vi "Example - Set Menu Items.vi"(8 "Error In":errorcluster, 10 "MenuHierarchyPaths":string[](array[string])=["Edit:Copy", "Edit:Paste", "Tools:Build", "Tools:Advanced:Mass Compile", "Tools:Advanced:Clear Cache"], 11 "Button":bool) -> (0 "Error Out":errorcluster)   [LabVIEW 2016, in "SLL Menu.lvlib"]
doc: "Example for Set Menu Items which builds a hierarchical run-time shortcut menu from colon-delimited paths."
uses:
  SLL Menu.lvlib
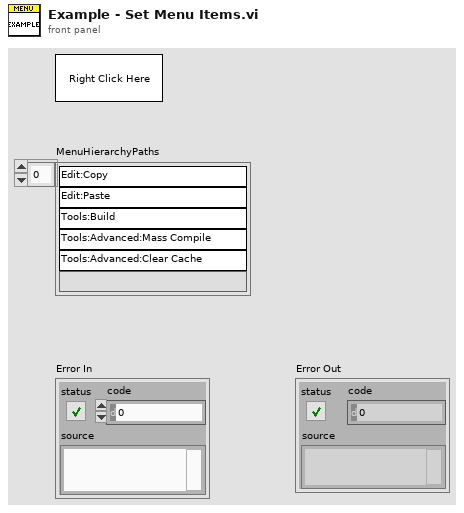
[diagram p1: front panel]
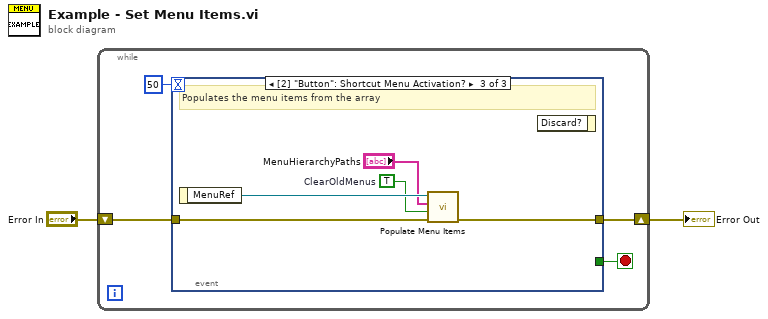
[diagram p0: block diagram]
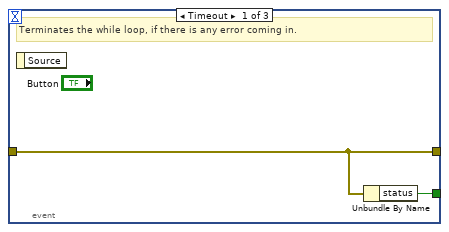
[diagram p2: hidden frame]
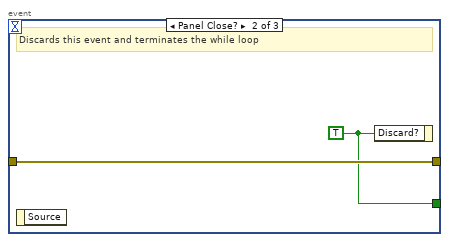
[diagram p3: hidden frame]
diagram:
  n1 = while {
    shift-right: [w3] -> w1
    shift-left: "Error In" -> [w4]
    stop <- w5 stop-if-true
    n2 = event shown="[2] \"Button\": Shortcut Menu Activation?" {
      selector: _ -> [_ _ _]
      dyn-events: _ -> [_ _ _]
      timeout: 50 -> [_ _ _]
      tunnel: [w7 w9 _] -> w5
      tunnel: w4 -> [w8 w10 w15]
      tunnel: [w8 w10 w13] -> w3
      event Timeout {
        # "Terminates the while loop, if there is any error coming in."
        n3 = event-data() -> ()  [unwired: 1 in, 1 out]
        n4 = Unbundle By Name(w8) -> ("status"=w7:bool)
      }
      event Panel Close? {
        w9 = TRUE ("Discard?")
        # "Discards this event and terminates the while loop"
        n5 = event-data() -> ()  [unwired: 1 in, 1 out]
        n6 = event-data("Discard?"=w9) -> ()  [unwired: 1 in, 1 out]
      }
      event "Button": Shortcut Menu Activation? {
        w11 = TRUE  # ClearOldMenus
        # "Populates the menu items from the array"
        n7 = event-data() -> ("MenuRef"=w14:refnum<k9>)  [unwired: 1 in]
        n8 = call "Populate Menu Items.vi"("Error In"=w15, "ClearOldMenus (T)"=w11, "MenuHierarchyPaths"="MenuHierarchyPaths", "MenuRef"=w14) -> ("Error Out"=w13:errorcluster)  [unwired: 7 in]
        n9 = event-data() -> ()  [unwired: 2 in, 1 out]
      }
    }
  }
  "Error Out" <- w1
